vi "NI6602_CreateTask.vi"(0 "task in":refnum<k21>, 1 "Camera Trigger":string="Dev1/ctr0", 2 "Exposure (s)":dbl=0.1 min=1.0 max=5000.0, 5 "Dye Settings":T1={"Dye Name"="", "Pulse Sequence"=[], "Emission Filter"=0, "Exposure (s)"=0.01, "Yellow Select"=FALSE, "# Pulses"=0} {"Exposure (s)" min=1.0 max=5000.0}, 7 "Sample Mode":T2(ring), 9 "Number of Samples":i32=100, 11 "error in":errorcluster) -> (4 "task out":refnum<k21>, 15 "error out":errorcluster)   [LabVIEW 2010]
uses:
  <vilib>/DAQmx/configure/trigger.llb/DAQmx Start Trigger (None).vi
  <vilib>/DAQmx/create/channels.llb/DAQmx Create Channel (CO-Pulse Generation-Time).vi
  <vilib>/DAQmx/configure/timing.llb/DAQmx Timing (Implicit).vi
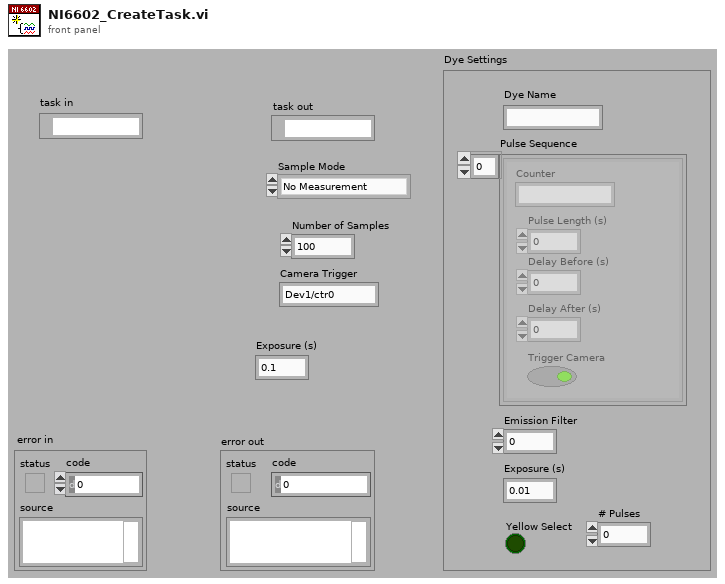
[diagram p1: front panel]
types:
  T1 = cluster{"Dye Name":string, "Pulse Sequence":cluster{"Counter":string, "Pulse Length (s)":dbl, "Delay Before (s)":dbl, "Delay After (s)":dbl, "Trigger Camera":bool}[], "Emission Filter":i16, "Exposure (s)":dbl, "Yellow Select":bool, "# Pulses":i32}
  T2 = enum16{"No Measurement", "Single Sample", "Continuous Samples", "N Samples"}
  T3 = cluster{"Counter":string, "Pulse Length (s)":dbl, "Delay Before (s)":dbl, "Delay After (s)":dbl, "Trigger Camera":bool}[]
  T4 = cluster{"Counter":string, "Pulse Length (s)":dbl, "Delay Before (s)":dbl, "Delay After (s)":dbl, "Trigger Camera":bool}
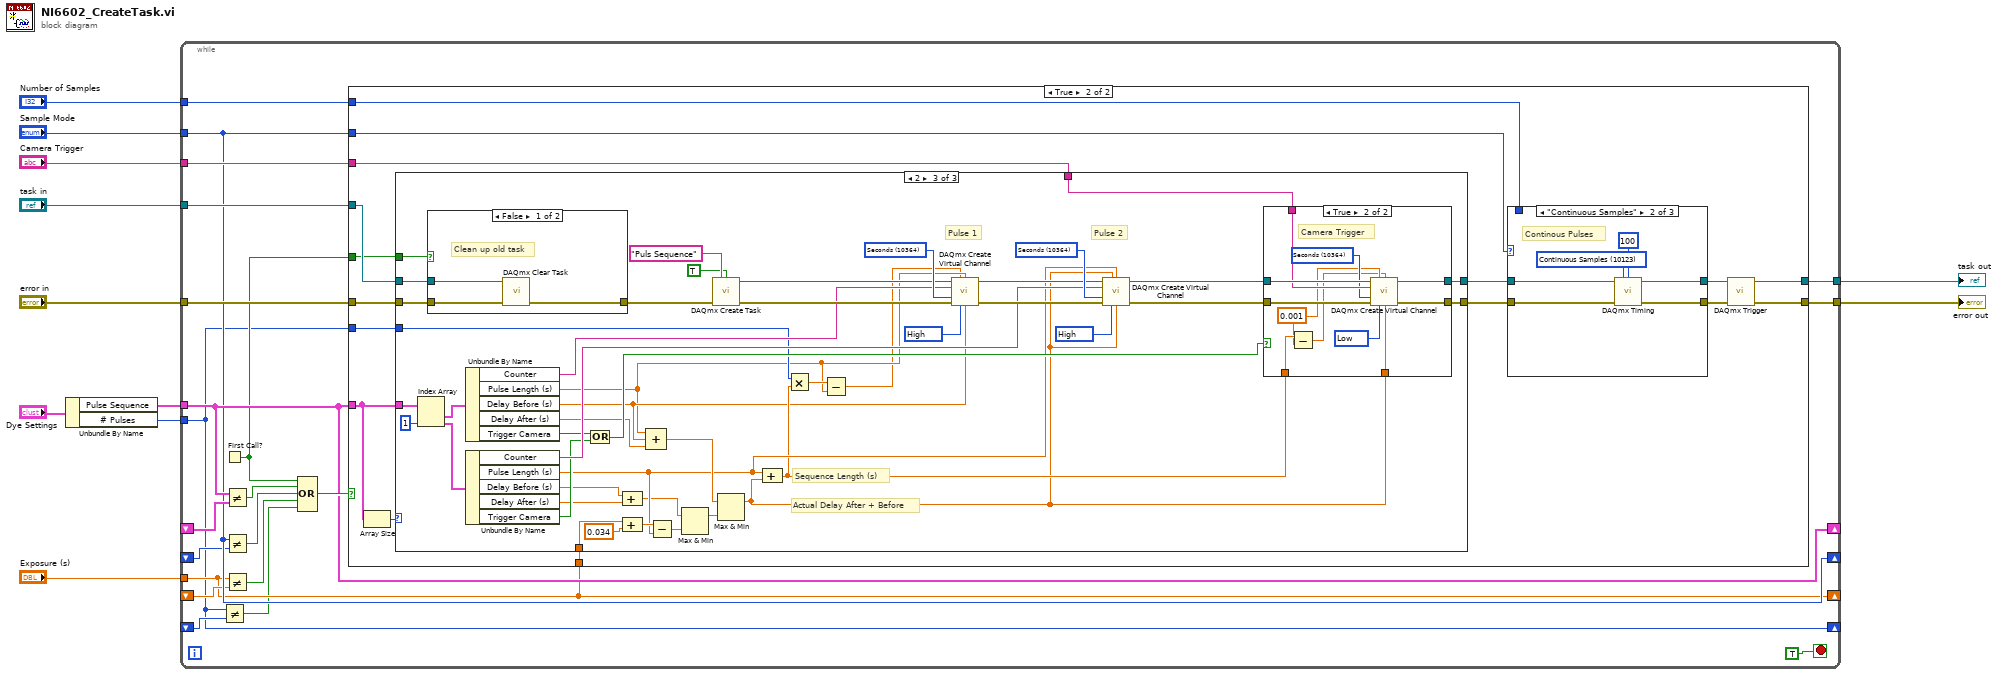
[diagram p0: block diagram]
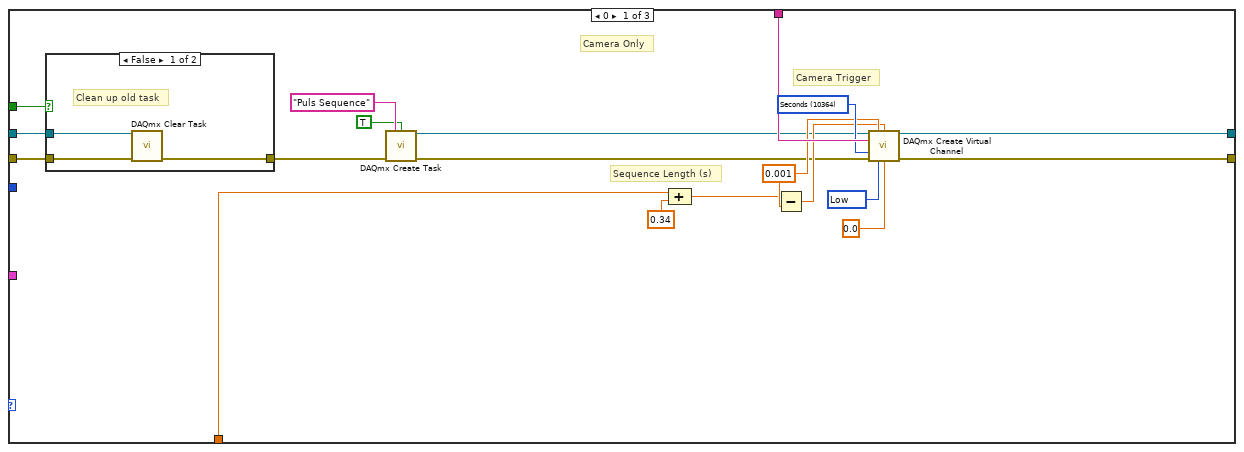
[diagram p3: hidden frame]
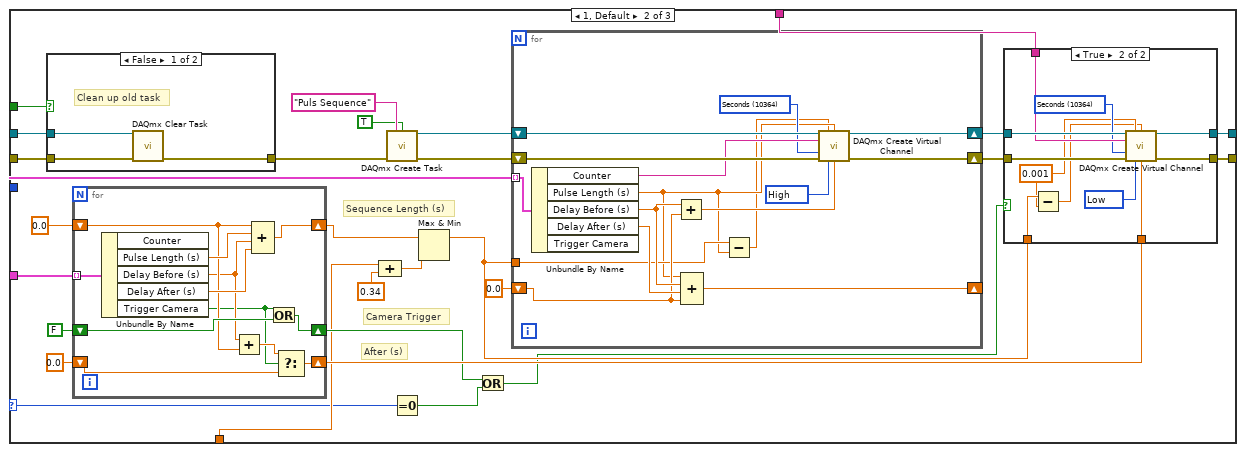
[diagram p5: hidden frame]
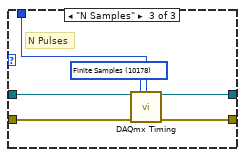
[diagram p11: hidden frame]
diagram:
  n1 = Unbundle By Name("Dye Settings") -> ("Pulse Sequence"=w2:T3, "# Pulses"=w1:i32)
  n2 = while {
    tunnel: w2 -> [w24]
    tunnel: "Number of Samples" -> [w30]
    tunnel: "Camera Trigger" -> [w29]
    tunnel: "Sample Mode" -> [w19]
    tunnel: "error in" -> [w27]
    tunnel: [w31] -> w10
    tunnel: [w32] -> w11
    shift-right: [w24] -> _
    shift-left: _ -> [w26]
    tunnel: "task in" -> [w23]
    shift-right: [w19] -> _
    shift-left: _ -> [w18]
    tunnel: "Exposure (s)" -> [w15]
    shift-right: [w15] -> _
    shift-left: _ -> [w16]
    tunnel: w1 -> [w12]
    shift-right: [w12] -> _
    shift-left: _ -> [w14]
    stop <- TRUE stop-if-true
    n3 = First Call?() -> (First Call?: T/F=w21:bool)
    n4 = Not Equal?(x=w12, y=w14) -> (x != y?=w13:bool)
    n5 = Not Equal?(x=w24, y=w26) -> (x != y?=w22:bool)
    n6 = Not Equal?(x=w19, y=w18) -> (x != y?=w20:bool)
    n7 = Not Equal?(x=w15, y=w16) -> (x != y?=w17:bool)
    n8 = Compound Arithmetic op=OR(w21, w22, w20, w17, w13) -> (w25:bool)
    n9 = case shown="True" w25 {
      tunnel: [w33 w48] -> w32
      tunnel: [w34 w47] -> w31
      tunnel: w30 -> [_ w46]
      tunnel: w29 -> [_ w43]
      tunnel: w19 -> [_ w42]
      tunnel: w27 -> [w34 w41]
      tunnel: w24 -> [_ w38]
      tunnel: w23 -> [w33 w40]
      tunnel: w21 -> [_ w39]
      tunnel: w15 -> [_ w37]
      tunnel: w12 -> [_ w35]
      frame False {
      }
      frame True {
        n10 = Array Size(array=w38) -> (size(s)=w36:i32)
        n11 = case shown="2" w36 {
          selector: w36 -> [_ w74 _]
          tunnel: [w67 w92 w189] -> w45
          tunnel: [w66 w90 w187] -> w44
          tunnel: w43 -> [w65 w89 w186]
          tunnel: w41 -> [w64 w88 w185]
          tunnel: w40 -> [w62 w86 w183]
          tunnel: w39 -> [w61 w85 w182]
          tunnel: w38 -> [_ w77 w177]
          tunnel: w37 -> [w59 w75 w180]
          tunnel: w35 -> [_ _ w155]
          frame 0 {
            w56 = 0.001 ("high time")
            w57 = 10214 items=["High"=10192, "Low"=10214] ("idle state")
            w58 = 10364 items=["Seconds"=10364] ("units")
            # "Camera Only"
            # "Camera Trigger"
            # "Sequence Length (s)"
            n12 = case shown="False" w61 {
              tunnel: w64 -> [w71 w73]
              tunnel: [w72 w73] -> w63
              tunnel: w62 -> [w70 _]
              frame False {
                # "Clean up old task"
                n13 = call <vilib>:"DAQmx Clear Task.vi"("task in"=w70, "error in"=w71) -> ("error out"=w72:errorcluster)  [unwired: 13 in]
              }
              frame True {
              }
            }
            n14 = call <vilib>:"DAQmx Create Task.vi"("new task name"="Puls Sequence", "auto cleanup"=TRUE, "error in"=w63) -> ("task out"=w53:refnum<k21>, "error out"=w54:errorcluster)  [unwired: 11 in]
            n15 = Compound Arithmetic op=ADD(w59, 0.34 ("Delay After (s) 2")) -> (w51:dbl)
            n16 = Subtract(x=w51, y=w56) -> (x-y=w55:dbl)
            n17 = call-poly <vilib>:"DAQmx Create Virtual Channel.vi"("task in"=w53, "high time"=w56, "low time"=w55, "counter"=w65, "units"=w58, "error in"=w54, "idle state"=w57, "initial delay"=0.0) -> ("task out"=w66:refnum<k21>, "error out"=w67:errorcluster)  [unwired: 6 in]
          }
          frame 1, Default {
            # "After (s)"
            # "Camera Trigger"
            # "Sequence Length (s)"
            n18 = case shown="False" w85 {
              tunnel: w88 -> [w103 w105]
              tunnel: [w104 w105] -> w87
              tunnel: w86 -> [w102 _]
              frame False {
                # "Clean up old task"
                n19 = call <vilib>:"DAQmx Clear Task.vi"("task in"=w102, "error in"=w103) -> ("error out"=w104:errorcluster)  [unwired: 13 in]
              }
              frame True {
              }
            }
            n20 = for {
              tunnel: w77 -> [w146] mode=indexing
              shift-right: [w143] -> w80
              shift-left: 0.0 -> [w139]
              shift-right: [w142] -> w79
              shift-left: FALSE -> [w141]
              shift-right: [w136] -> w81
              shift-left: 0.0 -> [w135]
              n21 = Unbundle By Name(w146) -> ("Pulse Length (s)"=w145:dbl, "Delay Before (s)"=w138:dbl, "Delay After (s)"=w144:dbl, "Trigger Camera"=w137:bool)  [unwired: 1 out]
              n22 = Add(x=w138, y=w139) -> (x+y=w140:dbl)
              n23 = Compound Arithmetic op=ADD(w139, w145, w138, w144) -> (w143:dbl)
              n24 = Or(x=w137, y=w141) -> (x .or. y?=w142:bool)
              n25 = Select(t=w140, s=w137, f=w135) -> (s? t:f=w136:dbl)
            }
            n26 = Compound Arithmetic op=ADD(w75, 0.34 ("Delay After (s) 2")) -> (w84:dbl)
            n27 = call <vilib>:"DAQmx Create Task.vi"("new task name"="Puls Sequence", "auto cleanup"=TRUE, "error in"=w87) -> ("task out"=w97:refnum<k21>, "error out"=w98:errorcluster)  [unwired: 11 in]
            n28 = Equal To 0?(x=w74) -> (x = 0?=w76:bool)
            n29 = Max & Min(x=w80, y=w84) -> (max(x,y)=w82:dbl)  [unwired: 1 out]
            n30 = Or(x=w79, y=w76) -> (x .or. y?=w78:bool)
            n31 = for {
              shift-right: [w131] -> w91
              shift-left: w97 -> [w132]
              shift-right: [w133] -> w93
              shift-left: w98 -> [w134]
              tunnel: w77 -> [w130] mode=indexing
              shift-right: [w127] -> _
              shift-left: 0.0 -> [w124]
              tunnel: w82 -> [w121]
              w122 = 10192 items=["High"=10192, "Low"=10214] ("idle state")
              w123 = 10364 items=["Seconds"=10364] ("units")
              n32 = Unbundle By Name(w130) -> ("Counter"=w129:string, "Pulse Length (s)"=w120:dbl, "Delay Before (s)"=w126:dbl, "Delay After (s)"=w128:dbl)  [unwired: 1 out]
              n33 = Add(x=w126, y=w124) -> (x+y=w125:dbl)
              n34 = Compound Arithmetic op=ADD(w120, w126, w128, w124) -> (w127:dbl)
              n35 = Subtract(x=w121, y=w120) -> (x-y=w119:dbl)
              n36 = call-poly <vilib>:"DAQmx Create Virtual Channel.vi"("task in"=w132, "high time"=w119, "low time"=w120, "counter"=w129, "units"=w123, "error in"=w134, "idle state"=w122, "initial delay"=w125) -> ("task out"=w131:refnum<k21>, "error out"=w133:errorcluster)  [unwired: 6 in]
            }
            n37 = case shown="True" w78 {
              tunnel: w93 -> [w107 w118]
              tunnel: [w107 w117] -> w92
              tunnel: w91 -> [w106 w116]
              tunnel: [w106 w115] -> w90
              tunnel: w89 -> [_ w114]
              tunnel: w81 -> [_ w111]
              tunnel: w82 -> [_ w110]
              frame False {
              }
              frame True {
                w109 = 0.001 ("high time")
                w112 = 10214 items=["High"=10192, "Low"=10214] ("idle state")
                w113 = 10364 items=["Seconds"=10364] ("units")
                n38 = Subtract(x=w110, y=w109) -> (x-y=w108:dbl)
                n39 = call-poly <vilib>:"DAQmx Create Virtual Channel.vi"("task in"=w116, "high time"=w109, "low time"=w108, "counter"=w114, "units"=w113, "error in"=w118, "idle state"=w112, "initial delay"=w111) -> ("task out"=w115:refnum<k21>, "error out"=w117:errorcluster)  [unwired: 6 in]
              }
            }
          }
          frame 2 {
            w172 = 10192 items=["High"=10192, "Low"=10214] ("idle state")
            w173 = 10364 items=["Seconds"=10364] ("units")
            w178 = 10192 items=["High"=10192, "Low"=10214] ("idle state")
            w179 = 10364 items=["Seconds"=10364] ("units")
            # "Actual Delay After + Before"
            # "Pulse 2"
            # "Pulse 1"
            # "Sequence Length (s)"
            n40 = Index Array(array=w177, index #2=1 ("index")) -> (element #1=w175:T4, element #2=w174:T4)  [unwired: 1 in]
            n41 = case shown="False" w182 {
              tunnel: w185 -> [w194 w196]
              tunnel: [w195 w196] -> w184
              tunnel: w183 -> [w193 _]
              frame False {
                # "Clean up old task"
                n42 = call <vilib>:"DAQmx Clear Task.vi"("task in"=w193, "error in"=w194) -> ("error out"=w195:errorcluster)  [unwired: 13 in]
              }
              frame True {
              }
            }
            n43 = Unbundle By Name(w175) -> ("Counter"=w167:string, "Pulse Length (s)"=w148:dbl, "Delay Before (s)"=w150:dbl, "Delay After (s)"=w158:dbl, "Trigger Camera"=w162:bool)
            n44 = Unbundle By Name(w174) -> ("Counter"=w166:string, "Pulse Length (s)"=w157:dbl, "Delay Before (s)"=w153:dbl, "Delay After (s)"=w154:dbl, "Trigger Camera"=w161:bool)
            n45 = Or(x=w162, y=w161) -> (x .or. y?=w160:bool)
            n46 = Compound Arithmetic op=ADD(w153, w154) -> (w152:dbl)
            n47 = Compound Arithmetic op=ADD(w180, 0.034 ("Delay After (s) 2")) -> (w159:dbl)
            n48 = Compound Arithmetic op=ADD(w148, w150, w158) -> (w163:dbl)
            n49 = Subtract(x=w159, y=w157) -> (x-y=w165:dbl)
            n50 = Max & Min(x=w152, y=w165) -> (max(x,y)=w164:dbl)  [unwired: 1 out]
            n51 = call <vilib>:"DAQmx Create Task.vi"("new task name"="Puls Sequence", "auto cleanup"=TRUE, "error in"=w184) -> ("task out"=w168:refnum<k21>, "error out"=w171:errorcluster)  [unwired: 11 in]
            n52 = Max & Min(x=w163, y=w164) -> (max(x,y)=w151:dbl)  [unwired: 1 out]
            n53 = Compound Arithmetic op=ADD(w157, w151) -> (w156:dbl)
            n54 = Multiply(x=w155, y=w156) -> (x*y=w149:dbl)
            n55 = Subtract(x=w149, y=w148) -> (x-y=w147:dbl)
            n56 = call-poly <vilib>:"DAQmx Create Virtual Channel.vi"("task in"=w168, "high time"=w147, "low time"=w148, "counter"=w167, "units"=w173, "error in"=w171, "idle state"=w172, "initial delay"=w150) -> ("task out"=w169:refnum<k21>, "error out"=w170:errorcluster)  [unwired: 6 in]
            n57 = call-poly <vilib>:"DAQmx Create Virtual Channel.vi"("task in"=w169, "high time"=w151, "low time"=w157, "counter"=w166, "units"=w179, "error in"=w170, "idle state"=w178, "initial delay"=w151) -> ("task out"=w188:refnum<k21>, "error out"=w190:errorcluster)  [unwired: 6 in]
            n58 = case shown="True" w160 {
              tunnel: w190 -> [w198 w209]
              tunnel: [w198 w208] -> w189
              tunnel: w188 -> [w197 w207]
              tunnel: [w197 w206] -> w187
              tunnel: w186 -> [_ w205]
              tunnel: w151 -> [_ w202]
              tunnel: w156 -> [_ w201]
              frame False {
              }
              frame True {
                w200 = 0.001 ("high time")
                w203 = 10214 items=["High"=10192, "Low"=10214] ("idle state")
                w204 = 10364 items=["Seconds"=10364] ("units")
                # "Camera Trigger"
                n59 = Subtract(x=w201, y=w200) -> (x-y=w199:dbl)
                n60 = call-poly <vilib>:"DAQmx Create Virtual Channel.vi"("task in"=w207, "high time"=w200, "low time"=w199, "counter"=w205, "units"=w204, "error in"=w209, "idle state"=w203, "initial delay"=w202) -> ("task out"=w206:refnum<k21>, "error out"=w208:errorcluster)  [unwired: 6 in]
              }
            }
          }
        }
        n61 = case shown="\"Continuous Samples\"" w42 {
          tunnel: w45 -> [w210 w217 w223]
          tunnel: [w210 w216 w222] -> w50
          tunnel: w44 -> [w211 w215 w221]
          tunnel: [w211 w214 w220] -> w49
          tunnel: w46 -> [_ _ w218]
          frame "Single Sample", Default {
          }
          frame "Continuous Samples" {
            w213 = 10123 items=["Finite Samples"=10178, "Continuous Samples"=10123, "Hardware Timed Single Point"=12522] ("sample mode")
            # "Continous Pulses"
            n62 = call-poly <vilib>:"DAQmx Timing.vi"("task/channels in"=w215, "sample mode"=w213, "samples per channel"=100, "error in"=w217) -> ("task out"=w214:refnum<k21>, "error out"=w216:errorcluster)  [unwired: 10 in]
          }
          frame "N Samples" {
            w219 = 10178 items=["Finite Samples"=10178, "Continuous Samples"=10123, "Hardware Timed Single Point"=12522] ("sample mode")
            # "N Pulses"
            n63 = call-poly <vilib>:"DAQmx Timing.vi"("task/channels in"=w221, "sample mode"=w219, "samples per channel"=w218, "error in"=w223) -> ("task out"=w220:refnum<k21>, "error out"=w222:errorcluster)  [unwired: 10 in]
          }
        }
        n64 = call-poly <vilib>:"DAQmx Trigger.vi"("task/channels in"=w49, "error in"=w50) -> ("task out"=w48:refnum<k21>, "error out"=w47:errorcluster)  [unwired: 12 in]
      }
    }
  }
  "task out" <- w11
  "error out" <- w10
